vi "与工控机交互(子VI).vi"   [LabVIEW 2016, in "数据传输系统.lvlib"]
uses:
  <vilib>/ptbypt/NI_PtbyPt.lvlib
types:
  T1 = cluster{"setini":string, "sysini":string, "hechaini":string, "actualwrite":string, "actualread":string, "datasent":string, "反控命令信息队列":string, "反控与仪器交互":string}
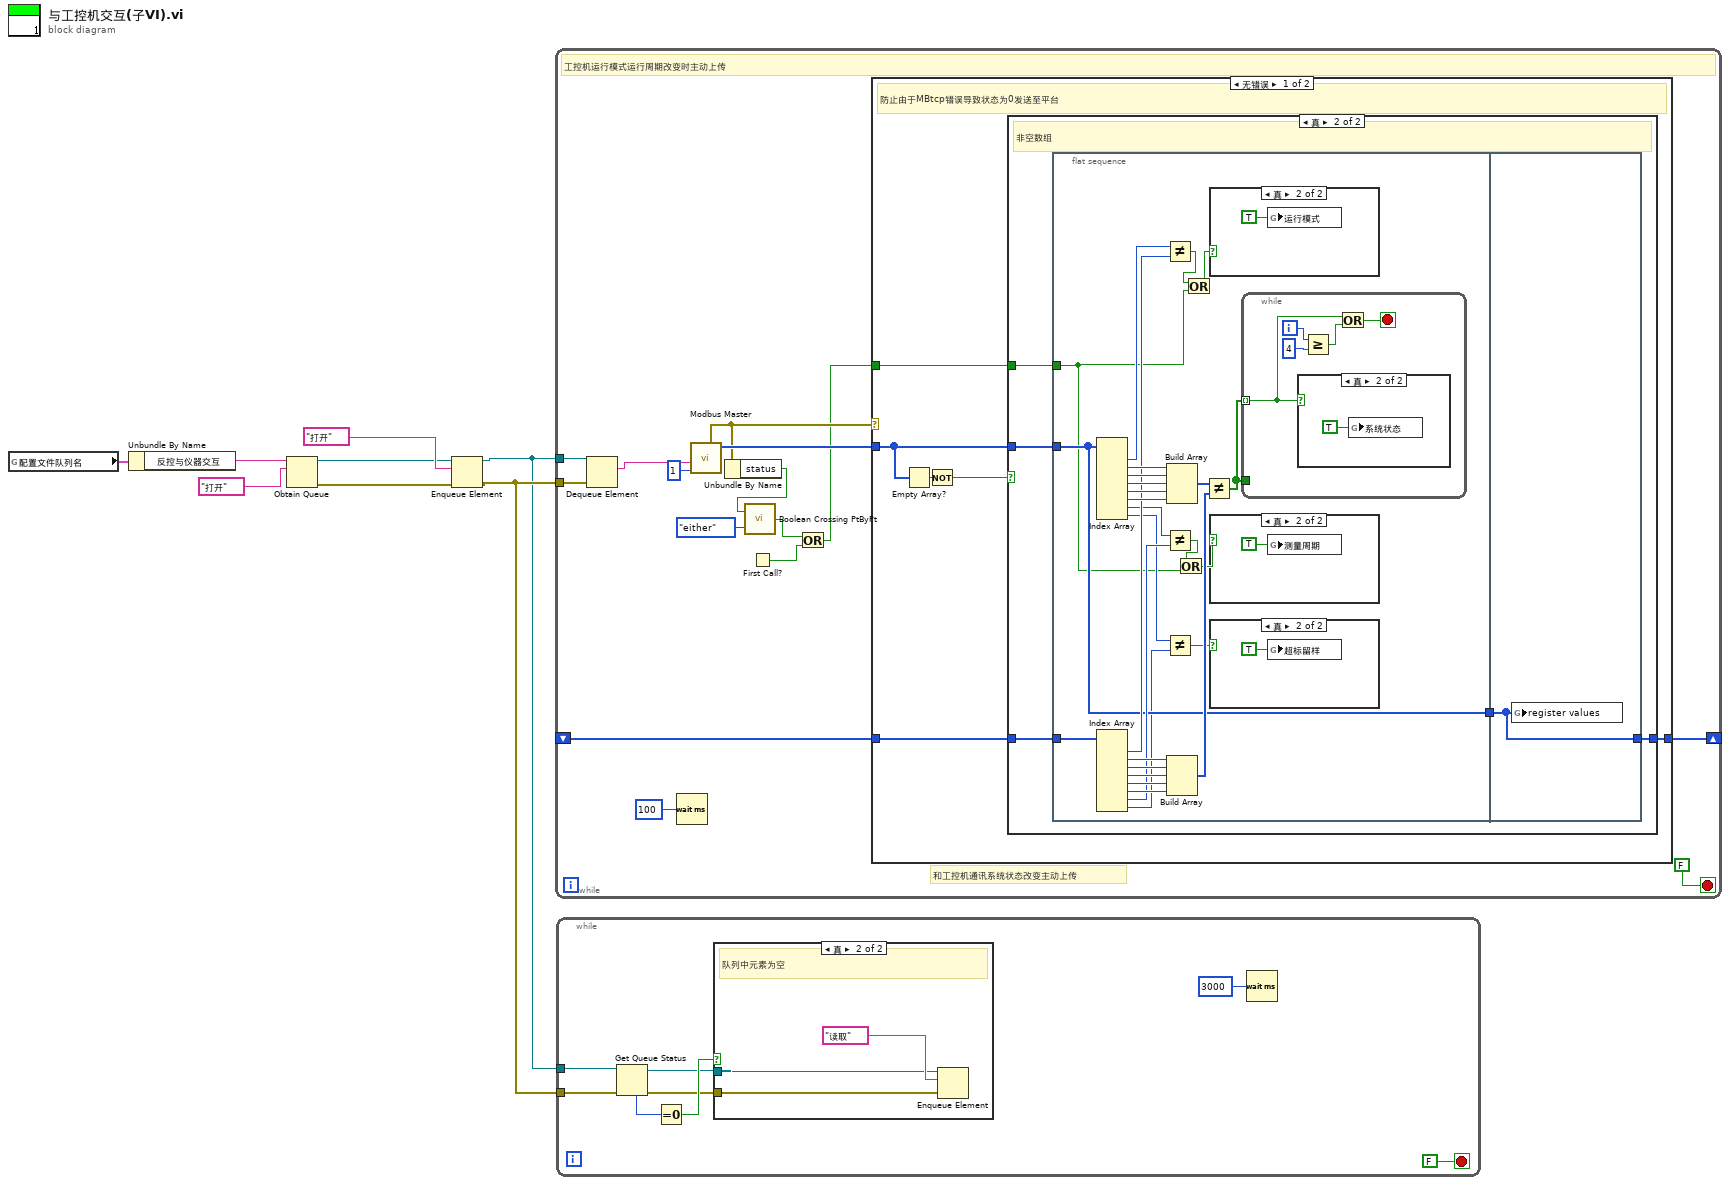
[diagram p0: block diagram]
diagram:
  n1 = global read "断电保存全局.vi" "配置文件队列名"() -> (w2:T1)
  n2 = Unbundle By Name(w2) -> ("反控与仪器交互"=w1:string)
  n3 = Obtain Queue(name (unnamed)=w1, element data type="打开" ("读取写入选择")) -> (queue out=w4:refnum<queue>, error out=w5:errorcluster)  [unwired: 3 in, 1 out]
  n4 = Enqueue Element(queue=w4, element="打开" ("读取写入选择"), error in (no error)=w5) -> (queue out=w6:refnum<queue>, error out=w7:errorcluster)  [unwired: 1 in, 1 out]
  n5 = while {
    tunnel: w6 -> [w19]
    tunnel: w7 -> [w18]
    shift-right: [w15] -> _
    shift-left: _ -> [w16]
    stop <- FALSE stop-if-true
    # "和工控机通讯系统状态改变主动上传"
    # "工控机运行模式运行周期改变时主动上传"
    n6 = Dequeue Element(queue=w19, error in (no error)=w18) -> (element=w17:string)  [unwired: 1 in, 3 out]
    n7 = Wait (ms)(milliseconds to wait=u32 100 ("等待时间（毫秒）")) -> ()  [unwired: 1 out]
    n8 = call "Modbus Master.vi"("Unit ID"=u8 1, "读取写入选择"=w17) -> ("register values"=w21:u16[], "error out"=w14:errorcluster)  [unwired: 8 in]
    n9 = Unbundle By Name(w14) -> ("status"=w13:bool)
    n10 = call <vilib>:"Boolean Crossing PtByPt.vi"("direction"=enum16{"either", "false-true", "true-false"}."either", "input"=w13) -> ("crossing"=w11:bool)  [unwired: 1 in]
    n11 = First Call?() -> (First Call?: T/F=w10:bool)
    n12 = Or(x=w11, y=w10) -> (x .or. y?=w9:bool)
    n13 = case shown="无错误" w14 {
      tunnel: w21 -> [w27 _]
      tunnel: w16 -> [w29 w73]
      tunnel: [w28 w73] -> w15
      tunnel: w9 -> [w24 _]
      frame No Error {
        # "防止由于MBtcp错误导致状态为0发送至平台"
        n14 = Empty Array?(array=w27) -> (empty?=w26:bool)
        n15 = Not(x=w26) -> (.not. x?=w25:bool)
        n16 = case shown="真" w25 {
          tunnel: w29 -> [w30 w34]
          tunnel: [w30 w33] -> w28
          tunnel: w27 -> [_ w32]
          tunnel: w24 -> [_ w31]
          frame False {
          }
          frame True {
            # "非空数组"
            n17 = flat-sequence {
              tunnel: w32 -> [w46]
              tunnel: [w46] -> w35
              tunnel: w34 -> [w42]
              tunnel: w31 -> [w37]
              tunnel: w35 -> [w72]
              tunnel: [w72] -> w33
              frame #0 {
                n18 = Index Array(array=w46) -> (element #1=w50:u16, element #2=w62:u16, element #3=w61:u16, element #4=w60:u16, element #5=w59:u16, element #6=w58:u16, element #7=w48:u16, element #8=w45:u16)  [unwired: 8 in]
                n19 = Index Array(array=w42) -> (element #1=w49:u16, element #2=w57:u16, element #3=w56:u16, element #4=w55:u16, element #5=w54:u16, element #6=w53:u16, element #7=w47:u16, element #8=w44:u16)  [unwired: 8 in]
                n20 = Not Equal?(x=w50, y=w49) -> (x != y?=w40:bool)
                n21 = Not Equal?(x=w48, y=w47) -> (x != y?=w38:bool)
                n22 = Not Equal?(x=w45, y=w44) -> (x != y?=w43:bool)
                n23 = Build Array(w62, w61, w60, w59, w58) -> (w52:u16[])
                n24 = Build Array(w57, w56, w55, w54, w53) -> (w51:u16[])
                n25 = Or(x=w38, y=w37) -> (x .or. y?=w36:bool)
                n26 = Or(x=w40, y=w37) -> (x .or. y?=w39:bool)
                n27 = Not Equal?(x=w52, y=w51) -> (x != y?=w41:bool[])
                n28 = case shown="真" w39 {
                  frame False {
                  }
                  frame True {
                    n29 = global write "全局1.vi" "运行模式"(TRUE) -> ()
                  }
                }
                n30 = case shown="真" w36 {
                  frame False {
                  }
                  frame True {
                    n31 = global write "全局1.vi" "测量周期"(TRUE ("系统状态改变")) -> ()
                  }
                }
                n32 = case shown="真" w43 {
                  frame False {
                  }
                  frame True {
                    n33 = global write "全局1.vi" "超标留样"(TRUE ("系统状态改变")) -> ()
                  }
                }
                n34 = while {
                  tunnel: w41 -> [w66] mode=indexing
                  tunnel: w41 -> [_]
                  i -> [w68]
                  stop <- w64 stop-if-true
                  n35 = case shown="真" w66 {
                    frame False {
                    }
                    frame True {
                      n36 = global write "全局1.vi" "系统状态"(TRUE ("系统状态改变")) -> ()
                    }
                  }
                  n37 = Greater Or Equal?(x=w68, y=4) -> (x >= y?=w65:bool)
                  n38 = Or(x=w66, y=w65) -> (x .or. y?=w64:bool)
                }
              }
              frame #1 {
                n39 = global write "全局1.vi" "register values"(w72) -> ()
              }
            }
          }
        }
      }
      frame Error {
      }
    }
  }
  n40 = while {
    tunnel: w6 -> [w78]
    tunnel: w7 -> [w77]
    stop <- FALSE stop-if-true
    n41 = Get Queue Status(queue=w78, error in (no error)=w77) -> (queue out=w75:refnum<queue>, error out=w74:errorcluster, # elements in queue=w79:i32)  [unwired: 1 in, 5 out]
    n42 = Equal To 0?(x=w79) -> (x = 0?=w76:bool)
    n43 = case shown="真" w76 {
      tunnel: w75 -> [_ w83]
      tunnel: w74 -> [_ w82]
      frame False {
      }
      frame True {
        # "队列中元素为空"
        n44 = Enqueue Element(queue=w83, element="读取" ("读取写入选择"), error in (no error)=w82) -> ()  [unwired: 1 in, 3 out]
      }
    }
    n45 = Wait (ms)(milliseconds to wait=u32 3000 ("等待时间（毫秒）")) -> ()  [unwired: 1 out]
  }
